vi "Boolean Stop After X or When Released.vi"(1 "Min Time Pressed":u64=1000, 2 "Go":bool) -> (0 "Output":bool)   [LabVIEW 2014]
panel:
  out "millisecond timer value":u32
  in  "Time To Go":u32
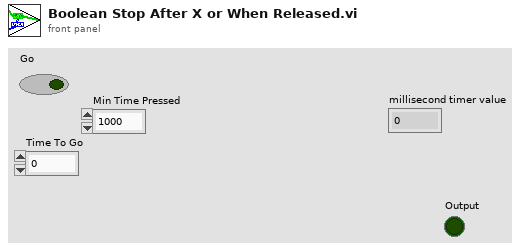
[diagram p1: front panel]
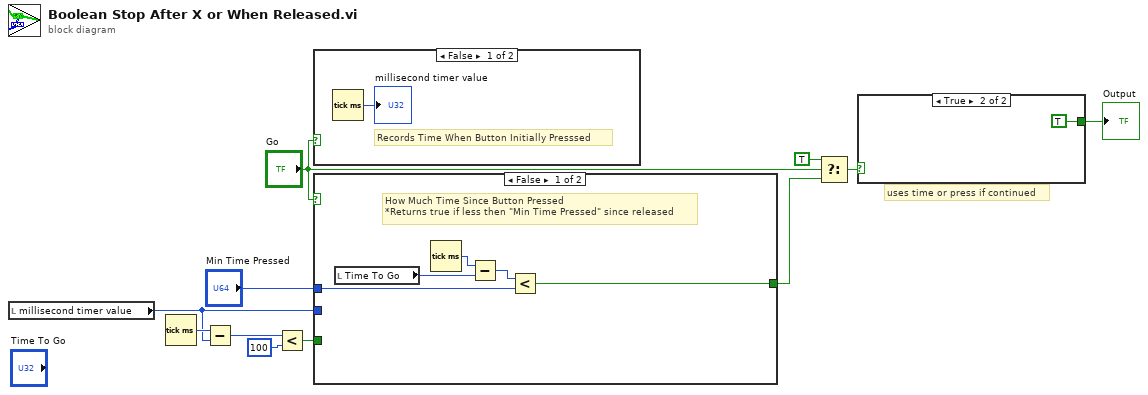
[diagram p0: block diagram]
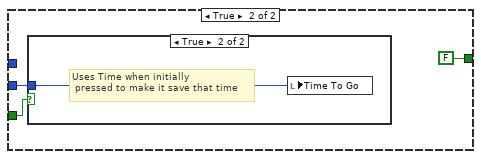
[diagram p3: hidden frame]
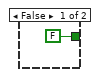
[diagram p5: hidden frame]
diagram:
  # "uses time or press if continued"
  n1 = local read "millisecond timer value"() -> (w1:u32)
  n2 = Tick Count (ms)() -> (millisecond timer value=w7:u32)
  n3 = Subtract(x=w7, y=w1) -> (x-y=w6:u32)
  n4 = Less?(x=w6, y=u32 100) -> (x < y?=w4:bool)
  n5 = case shown="False" "Go" {
    frame False {
      # "Records Time When Button Initially Presssed"
      n6 = Tick Count (ms)() -> (millisecond timer value=→"millisecond timer value":u32)
    }
    frame True {
    }
  }
  n7 = case shown="False" "Go" {
    tunnel: "Min Time Pressed" -> [w14 _]
    tunnel: [w13 FALSE] -> w8
    tunnel: w4 -> [_ w19]
    tunnel: w1 -> [_ w18]
    frame False {
      # "How Much Time Since Button Pressed\n*Returns true if less then \"Min Time Pressed\" since released"
      n8 = local read "Time To Go"() -> (w16:u32)
      n9 = Tick Count (ms)() -> (millisecond timer value=w15:u32)
      n10 = Subtract(x=w15, y=w16) -> (x-y=w17:u32)
      n11 = Less?(x=w17, y=w14) -> (x < y?=w13:bool)
    }
    frame True {
      n12 = case shown="True" w19 {
        tunnel: w18 -> [_ w21]
        frame False {
        }
        frame True {
          # "Uses Time when initially\n pressed to make it save that time"
          n13 = local write "Time To Go"(w21) -> ()
        }
      }
    }
  }
  n14 = Select(t=TRUE, s="Go", f=w8) -> (s? t:f=w10:bool)
  n15 = case shown="True" w10 {
    tunnel: [FALSE TRUE] -> w2
    frame False {
    }
    frame True {
    }
  }
  "Output" <- w2
